vi "Agilent U2722 - DC Power Output DC Volts1.vi"() -> ()   [LabVIEW 2010]
doc: "This example shows how to configure the instrument's output voltage level, over current protection, and over voltage protection. The actual voltage level and actual current level are returned as well as whether over voltage protection (OVP) or over current protection (OCP) has been tripped."
uses:
  Public/Configure/Configure Channel (Voltage).vi
  Agilent U2722.lvlib
panel:
  in  "Voltage Range (0: 2 Volts)":u16(ring) items=["2 Volts", "20 Volts"]
  in  "Current Limit":dbl=2.0
  in  "Output Level (V)":dbl=1.0
  in  "Channel (1: Channel 1)":u16(ring)=1 items=["Channel 1"=1, "Channel 2"=2, "Channel 3"=3]
  in  "Stop Output":bool
  out "Actual Current Limit (A)":dbl format="%.2f"
  out "Actual Voltage Level (V)":dbl format="%.2f"
  in  "VISA resource name":refnum<visa-resource-name>
  # "(c) 2009 National Instruments.  ALL RIGHTS RESERVED."
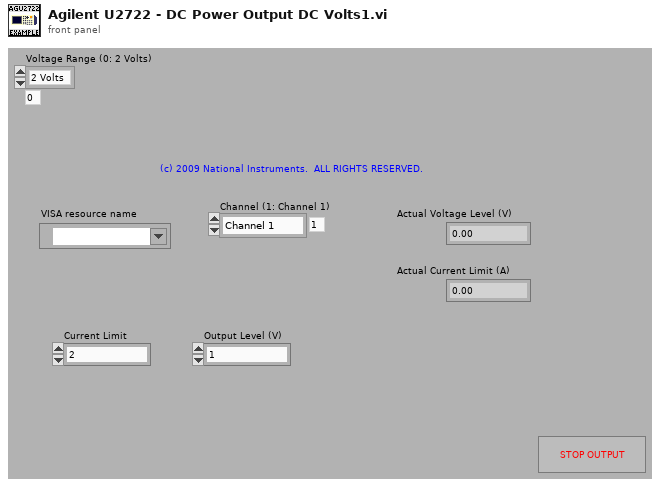
[diagram p1: front panel]
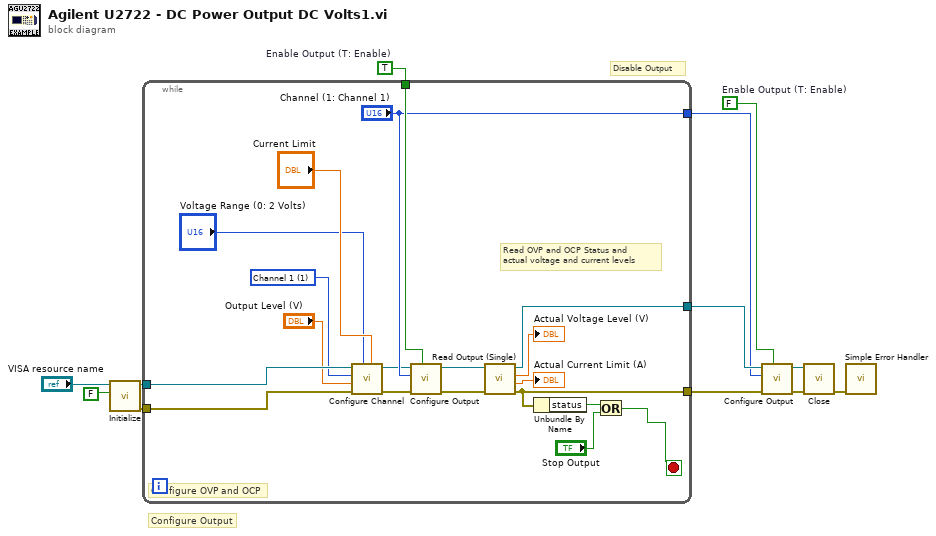
[diagram p0: block diagram]
diagram:
  w10 = TRUE  # Enable Output (T: Enable)
  w5 = FALSE  # Enable Output (T: Enable)
  # "Disable Output"
  # "Configure Output"
  n1 = call "Initialize.vi"("ID Query (True)"=FALSE, "VISA resource name"="VISA resource name") -> ("error out"=w1:errorcluster, "VISA resource name out"=w2:refnum<visa-resource-name>)  [unwired: 8 in]
  n2 = while {
    tunnel: w10 -> [w31]
    tunnel: [w28] -> w9
    tunnel: [w27] -> w8
    tunnel: ["Channel (1: Channel 1)"] -> w4
    tunnel: w2 -> [w25]
    tunnel: w1 -> [w24]
    stop <- w14 stop-if-true
    w21 = u16 1 items=["Channel 1"=1, "Channel 2"=2, "Channel 3"=3] ("Channel (1: Channel 1)")
    # "Read OVP and OCP Status and\nactual voltage and current levels"
    # "Configure OVP and OCP"
    n3 = call-poly "Configure Channel.vi"("Current Limit (1.0 uA)"="Current Limit", "Voltage Range (0: 2 Volts)"="Voltage Range (0: 2 Volts)", "error in (no error)"=w24, "Output Level (1.0 V)"="Output Level (V)", "Channel (1: Channel 1)"=w21, "VISA resource name"=w25) -> ("error out"=w22:errorcluster, "VISA resource name out"=w23:refnum<visa-resource-name>)  [unwired: 4 in]
    n4 = call "Configure Output.vi"("Enable Output (T: Enable)"=w31, "error in (no error)"=w22, "Channel (1: Channel 1)"="Channel (1: Channel 1)", "VISA resource name"=w23) -> ("error out"=w29:errorcluster, "VISA resource name out"=w30:refnum<visa-resource-name>)  [unwired: 6 in]
    n5 = call "Read Output (Single).vi"("error in (no error)"=w29, "VISA resource name"=w30) -> ("error out"=w27:errorcluster, "Actual Current Level (A)"=→"Actual Current Limit (A)":dbl, "Actual Voltage Level (V)"=→"Actual Voltage Level (V)":dbl, "VISA resource name out"=w28:refnum<visa-resource-name>)  [unwired: 6 in]
    n6 = Unbundle By Name(w27) -> ("status"=w15:bool)
    n7 = Or(x=w15, y="Stop Output") -> (x .or. y?=w14:bool)
  }
  n8 = call "Configure Output.vi"("Enable Output (T: Enable)"=w5, "error in (no error)"=w8, "Channel (1: Channel 1)"=w4, "VISA resource name"=w9) -> ("error out"=w6:errorcluster, "VISA resource name out"=w7:refnum<visa-resource-name>)  [unwired: 6 in]
  n9 = call "Close.vi"("error in (no error)"=w6, "VISA resource name"=w7) -> ("error out"=w12:errorcluster)  [unwired: 9 in]
  n10 = call <vilib>:"Simple Error Handler.vi"("error in (no error)"=w12) -> ()  [unwired: 4 in, 5 out]
